vi "MotorControllerFollow.vi"(5 "LeaderConfig":T1={"CAN Address"=0, "Invert"=FALSE, "InvertSensor"=FALSE, "Unit Conversion Factor"=0.0, "Brake Mode"=enum."Override to Brake", "Reverse Limt Switch Mode"=enum."Disabled", "Forward Limt Swith Mode"=enum."Disabled", "PWM Channel"=enum."Invalid", "Motor Controller Type"=enum."Talon SRX", "Peak Current (A)"=0, "Continuous Current (A)"=0, "Peak Duration (ms)"=0, "Current Limit Enable"=FALSE}, 7 "FollowerConfig":T1={"CAN Address"=0, "Invert"=FALSE, "InvertSensor"=FALSE, "Unit Conversion Factor"=0.0, "Brake Mode"=enum."Override to Brake", "Reverse Limt Switch Mode"=enum."Disabled", "Forward Limt Swith Mode"=enum."Disabled", "PWM Channel"=enum."Invalid", "Motor Controller Type"=enum."Talon SRX", "Peak Current (A)"=0, "Continuous Current (A)"=0, "Peak Duration (ms)"=0, "Current Limit Enable"=FALSE}, 8 "error in (no error)":errorcluster, 10 "LeaderDevRef":T6, 11 "FollowerDevRef":T6) -> (0 "error out":errorcluster, 3 "FollowerDevRefOut":T6)   [LabVIEW 2019, in "ArgosLib.lvlib"]
uses:
  ArgosLib.lvlib
  <vilib>/Rock Robotics/WPI/MotorControl/WPI_MotorControlDeviceRef.ctl
  <vilib>/Rock Robotics/WPI/MotorControl/WPI_MotorControlType.ctl
  <vilib>/Rock Robotics/SystemInterfaces/DIO/FPGA_DIOPWMChannel.ctl
  <vilib>/Rock Robotics/WPI/PWM/WPI_PWMDeadband.ctl
  <vilib>/Rock Robotics/SystemInterfaces/DIO/FPGA_DIOChannel.ctl
  Config/ConfigComponents/TypeDefs/Config_Motor.ctl
  <vilib>/Rock Robotics/WPI/ThirdParty/Phoenix-LabVIEW/Motor Controller/Controls/CTRE_Phoenix_MotorControl_NeutralMode.ctl
  <vilib>/Rock Robotics/WPI/ThirdParty/Phoenix-LabVIEW/Motor Controller/Controls/CTRE_Phoenix_MotorControl_LimitSwitchNormal.ctl
  Config/ConfigComponents/TypeDefs/Config_MotorCtrlType.ctl
  <vilib>/Playing With Fusion Inc/Playing With Fusion Lib for FRC/PWF_Venom_LabVIEW/PwF_Venom.lvlib
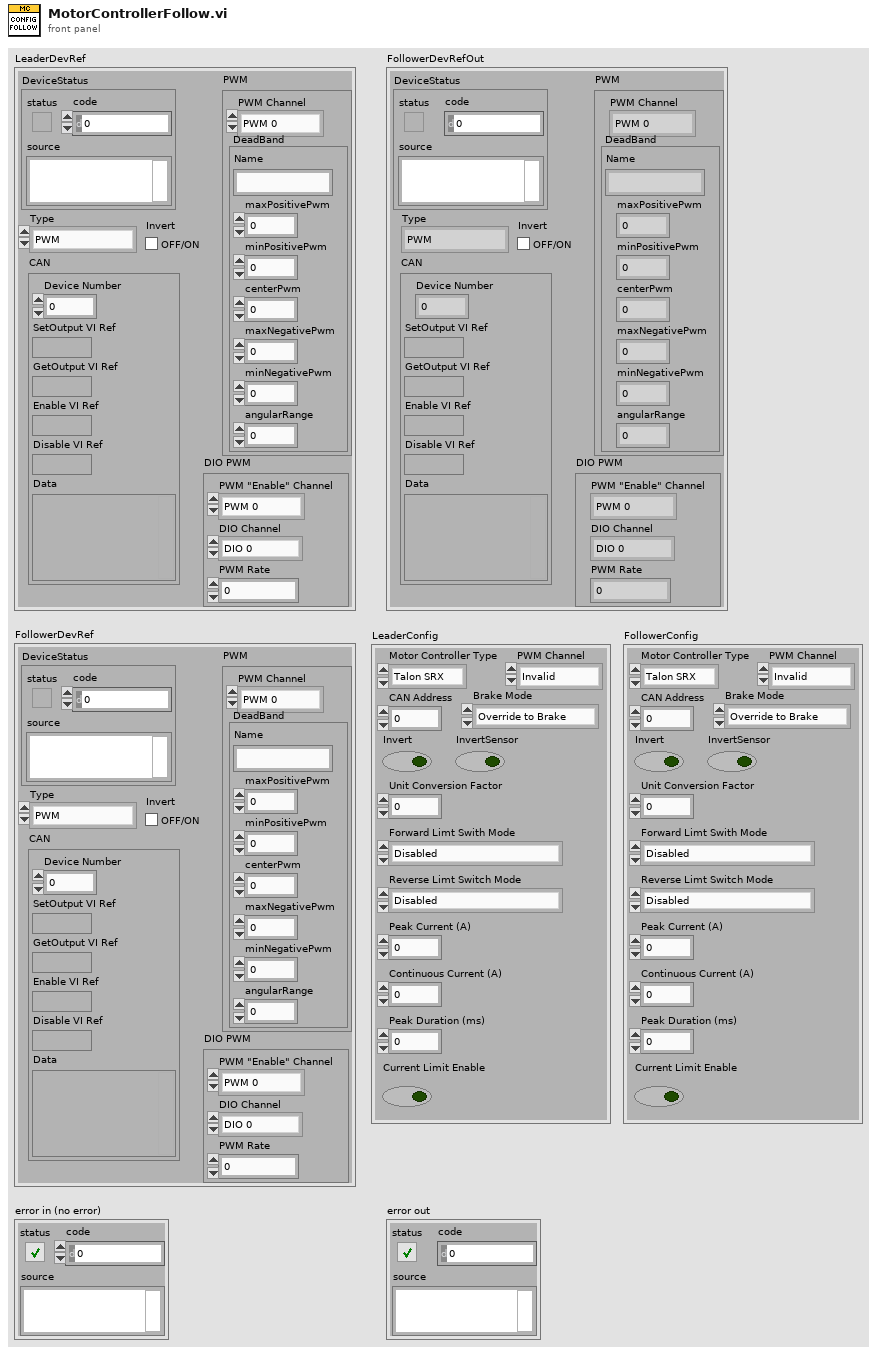
[diagram p1: front panel]
types:
  T1 = typedef "ArgosLib.lvlib/Config_Motor.ctl" = cluster{"CAN Address":u8, "Invert":bool, "InvertSensor":bool, "Unit Conversion Factor":dbl, "Brake Mode":T2, "Reverse Limt Switch Mode":T3, "Forward Limt Swith Mode":T3, "PWM Channel":T4, "Motor Controller Type":T5, "Peak Current (A)":i32, "Continuous Current (A)":i32, "Peak Duration (ms)":i32, "Current Limit Enable":bool}
  T2 = typedef "CTRE_Phoenix_MotorControl_NeutralMode.ctl" = enum8{"EEPROMSetting", "Override to Coast", "Override to Brake"}
  T3 = typedef "CTRE_Phoenix_MotorControl_LimitSwitchNormal.ctl" = enum16{"Normally Open", "Normally Closed", "Disabled"}
  T4 = typedef "FPGA_DIOPWMChannel.ctl" = enum8{"PWM 0", "PWM 1", "PWM 2", "PWM 3", "PWM 4", "PWM 5", "PWM 6", "PWM 7", "PWM 8", "PWM 9", "PWM MXP 0", "PWM MXP 1", "PWM MXP 2", "PWM MXP 3", "PWM MXP 4", "PWM MXP 5", "PWM MXP 6", "PWM MXP 7", "PWM MXP 8", "PWM MXP 9", "Invalid"}
  T5 = typedef "ArgosLib.lvlib/Config_MotorCtrlType.ctl" = enum16{"Disabled", "Talon SRX", "Talon SR", "Venom", "Spark MAX", "Falcon FX"}
  T6 = typedef "WPI_MotorControlDeviceRef.ctl" = cluster{"DeviceStatus":errorcluster, "Type":T7, "PWM":cluster{"PWM Channel":T4, "DeadBand":T8}, "CAN":cluster{"Device Number":u8, "SetOutput VI Ref":variant, "GetOutput VI Ref":variant, "Enable VI Ref":variant, "Disable VI Ref":variant, "Data":variant}, "Invert":bool, "DIO PWM":cluster{"PWM \"Enable\" Channel":T4, "DIOChannel":T9, "PWM Rate":dbl}}
  T7 = typedef "WPI_MotorControlType.ctl" = enum16{"PWM", "CAN", "DIO PWM"}
  T8 = typedef "WPI_PWMDeadband.ctl" = cluster{"Name":string, "maxPositivePwm":i32, "minPositivePwm":i32, "centerPwm":i32, "maxNegativePwm":i32, "minNegativePwm":i32, "angularRange":u16}
  T9 = typedef "FPGA_DIOChannel.ctl" = enum8{"DIO 0", "DIO 1", "DIO 2", "DIO 3", "DIO 4", "DIO 5", "DIO 6", "DIO 7", "DIO 8", "DIO 9", "DIO MXP 0", "DIO MXP 1", "DIO MXP 2", "DIO MXP 3", "DIO MXP 4", "DIO MXP 5", "DIO MXP 6", "DIO MXP 7", "DIO MXP 8", "DIO MXP 9", "DIO MXP 10", "DIO MXP 11", "DIO MXP 12", "DIO MXP 13", "DIO MXP 14", "DIO MXP 15", "SPI Port CS1", "SPI Port CS2", "SPI Port CS3", "SPI Port MISO", "SPI Port MOSI", "Invalid"}
  T10 = enum16{"FollowerType_PercentOutput", "FollowerType_AuxOutput1"}
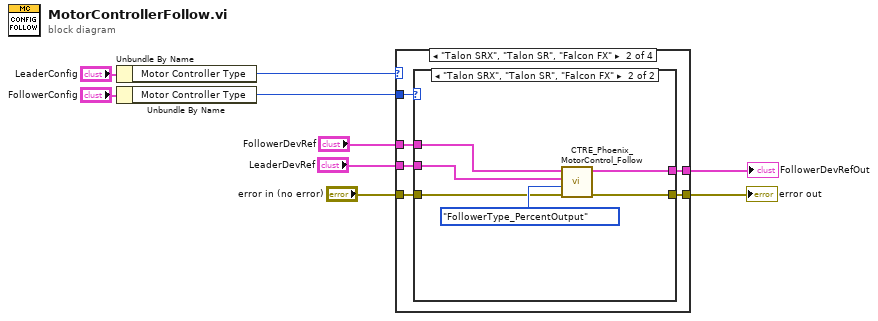
[diagram p0: block diagram]
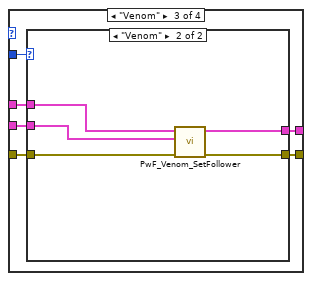
[diagram p4: hidden frame]
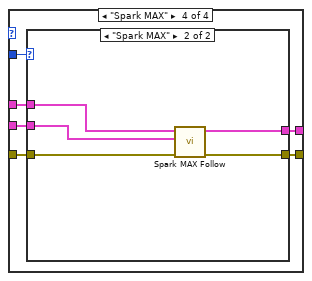
[diagram p6: hidden frame]
diagram:
  n1 = Unbundle By Name("LeaderConfig") -> ("Motor Controller Type"=w2:T5)
  n2 = Unbundle By Name("FollowerConfig") -> ("Motor Controller Type"=w1:T5)
  n3 = case shown="\"Talon SRX\", \"Talon SR\", \"Falcon FX\"" w2 {
    tunnel: [w10 w17 w31 w44] -> w9
    tunnel: "error in (no error)" -> [w10 w16 w30 w43]
    tunnel: "LeaderDevRef" -> [_ w15 w29 w42]
    tunnel: "FollowerDevRef" -> [w11 w14 w28 w41]
    tunnel: [w11 w13 w27 w40] -> w5
    tunnel: w1 -> [_ w12 w26 w39]
    frame "Disabled", Default {
    }
    frame "Talon SRX", "Talon SR", "Falcon FX" {
      n4 = case shown="\"Talon SRX\", \"Talon SR\", \"Falcon FX\"" w12 {
        tunnel: [w18 w24] -> w17
        tunnel: w16 -> [w18 w23]
        tunnel: w15 -> [_ w22]
        tunnel: w14 -> [w19 w21]
        tunnel: [w19 w20] -> w13
        frame "Disabled", Default {
        }
        frame "Talon SRX", "Talon SR", "Falcon FX" {
          n5 = call <vilib>:"CTRE_Phoenix_MotorControl_Follow.vi"("error in (no error)"=w23, "FollowerType"=T10."FollowerType_PercentOutput", "Master Controller to Follow"=w22, "PhoenixMotorControlDevRef"=w21) -> ("error out"=w24:errorcluster, "PhoenixMotorControlDevRef"=w20:T6)  [unwired: 6 in]
        }
      }
    }
    frame "Venom" {
      n6 = case shown="\"Venom\"" w26 {
        tunnel: [w32 w38] -> w31
        tunnel: w30 -> [w32 w37]
        tunnel: w29 -> [_ w36]
        tunnel: w28 -> [w33 w35]
        tunnel: [w33 w34] -> w27
        frame "Disabled", Default {
        }
        frame "Venom" {
          n7 = call <vilib>:"PwF_Venom_SetFollower.vi"("error in"=w37, "LeaderDevRef"=w36, "PwFVenomDevRefIn"=w35) -> ("error out"=w38:errorcluster, "PwFVenomDevRefOut"=w34:T6)  [unwired: 7 in]
        }
      }
    }
    frame "Spark MAX" {
      n8 = case shown="\"Spark MAX\"" w39 {
        tunnel: [w45 w51] -> w44
        tunnel: w43 -> [w45 w50]
        tunnel: w42 -> [_ w49]
        tunnel: w41 -> [w46 w48]
        tunnel: [w46 w47] -> w40
        frame "Disabled", Default {
        }
        frame "Spark MAX" {
          n9 = call <vilib>:"Spark MAX Follow.vi"("error in (no error)"=w50, "Master Controller"=w49, "MotorControlDeviceRef"=w48) -> ("error out"=w51:errorcluster, "MotorControlDeviceRef"=w47:T6)  [unwired: 7 in]
        }
      }
    }
  }
  "error out" <- w9
  "FollowerDevRefOut" <- w5
